vi "Session Reservation Json to Data Cluster.vi"(8 "error in":errorcluster, 11 "json in":string) -> (0 "error out":errorcluster, 3 "data out":T1)   [LabVIEW 2020, in "MeasurementServerTests.lvlib"]
uses:
  MeasurementServerTests.lvlib
  Runtime/MeasurementLink Session Management/Session Reservation/Data.ctl
  Runtime/MeasurementLink Session Management/Connection Map/Connection Map.lvclass
  Runtime/MeasurementLink Session Management/Session Reservation/Session and Driver Info.ctl
  Runtime/MeasurementLink Session Management Client/RPC Messages/ni_measurementlink_sessionmanagement_v1_SessionInformation.ctl
  Runtime/MeasurementLink Session Management Client/RPC Messages/nidevice_grpc_Session.ctl
  Runtime/MeasurementLink Session Management Client/RPC Messages/ni_measurementlink_sessionmanagement_v1_ChannelMapping.ctl
  Runtime/MeasurementLink Session Management Client/RPC Messages/ni_measurementlink_PinMapContext.ctl
  2dfce5ba-96f1-4d0e-9517-3e25601897e8.vi
  <vilib>/JDP Science/JSONtext/JSON text to Variant.vi
  <vilib>/JDP Science/JSONtext/LVClass Serializer/JSONtext LVClass Serializer.lvclass
  Runtime/MeasurementLink Session Management/Session Reservation/Session Reservation.lvclass
  Runtime/MeasurementLink Session Management Client/MeasurementLink Session Management Client.lvlib
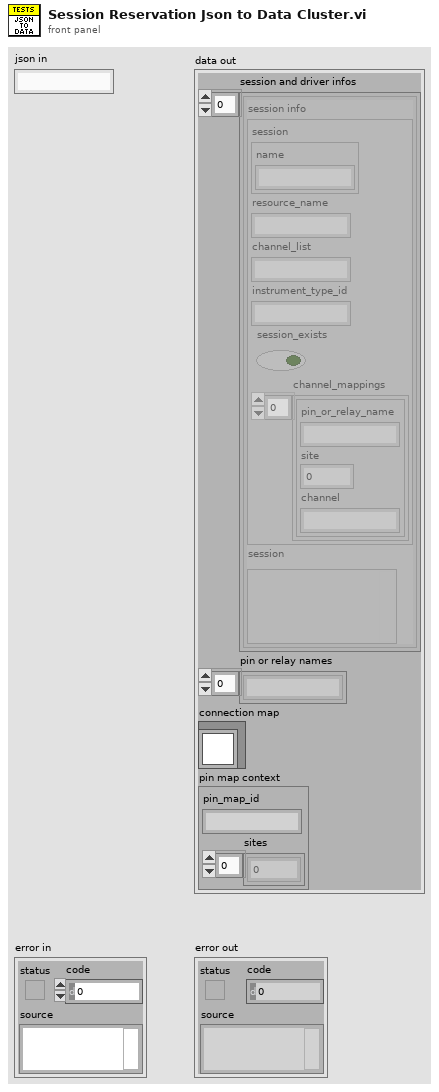
[diagram p1: front panel]
types:
  T1 = typedef "MeasurementLink Session Management.lvlib/Session Reservation.lvclass/Data.ctl" = cluster{"session and driver infos":T2[], "pin or relay names":string[], "connection map":refnum<class "Connection Map.lvclass">, "pin map context":T6}
  T2 = typedef "MeasurementLink Session Management.lvlib/Session Reservation.lvclass/Session and Driver Info.ctl" = cluster{"session info":T3, "session":variant}
  T3 = typedef "MeasurementLink Session Management Client.lvlib/ni_measurementlink_sessionmanagement_v1_SessionInformation.ctl" = cluster{"session":T4, "resource_name":string, "channel_list":string, "instrument_type_id":string, "session_exists":bool, "channel_mappings":T5[]}
  T4 = typedef "MeasurementLink Session Management Client.lvlib/nidevice_grpc_Session.ctl" = cluster{"name":string}
  T5 = typedef "MeasurementLink Session Management Client.lvlib/ni_measurementlink_sessionmanagement_v1_ChannelMapping.ctl" = cluster{"pin_or_relay_name":string, "site":i32, "channel":string}
  T6 = typedef "MeasurementLink Session Management Client.lvlib/ni_measurementlink_PinMapContext.ctl" = cluster{"pin_map_id":string, "sites":i32[]}
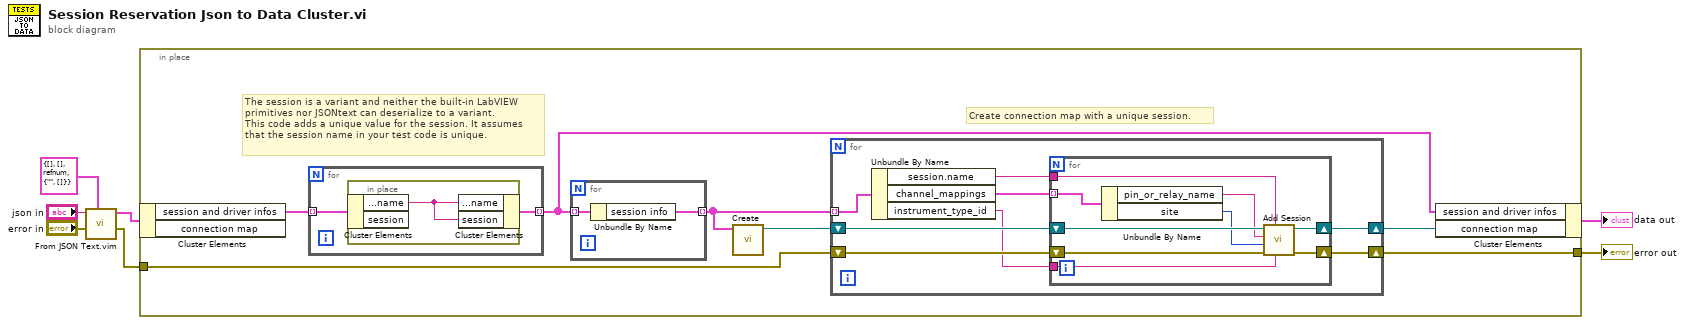
[diagram p0: block diagram]
diagram:
  n1 = call "From JSON Text.vim"("Data Type and Default Value"=T1 {"session and driver infos"=[], "pin or relay names"=[], "connection map"=refnum, "pin map context"={"pin_map_id"="", "sites"=[]}} ("data"), "error in (no error)"="error in", "JSON"="json in") -> ("error out"=w2:errorcluster, "Data out"=w5:T1)  [unwired: 7 in]
  n2 = in-place {
    in-place-border: w2 -> [w12]
    in-place-border: [w11] -> w1
    # "Create connection map with a unique session."
    # "The session is a variant and neither the built-in LabVIEW\nprimitives nor JSONtext can deserialize to a variant.\nThis code adds a unique value for the session. It assumes\nthat the session name in your test code is unique."
    n3 = in-place-cluster #1(w5) -> ("session and driver infos"=w9:T2[])  [unwired: 1 out]
    n4 = for {
      tunnel: w9 -> [w16] mode=indexing
      tunnel: [w15] -> w8 mode=indexing
      n5 = in-place {
        n6 = in-place-cluster #2(w16) -> ("session info.session.name"=w17:string)  [unwired: 1 out]
        n7 = in-place-cluster #2("session info.session.name"=w17, "session"=w17) -> (w15:T2)
      }
    }
    n8 = for {
      tunnel: w8 -> [w36] mode=indexing
      tunnel: [w35] -> w10 mode=indexing
      n9 = Unbundle By Name(w36) -> ("session info"=w35:T3)
    }
    n10 = call "Create.vi"("session info"=w10) -> ("connection map"=w14:refnum<class "Connection Map.lvclass">)  [unwired: 10 in]
    n11 = for {
      shift-right: [w24] -> w13
      shift-left: w14 -> [w25]
      shift-right: [w22] -> w11
      shift-left: w12 -> [w23]
      tunnel: w10 -> [w21] mode=indexing
      n12 = Unbundle By Name(w21) -> ("session.name"=w18:string, "channel_mappings"=w20:T5[], "instrument_type_id"=w19:string)
      n13 = for {
        shift-right: [w33] -> w24
        shift-left: w25 -> [w34]
        shift-right: [w31] -> w22
        shift-left: w23 -> [w32]
        tunnel: w20 -> [w30] mode=indexing
        tunnel: w19 -> [w27]
        tunnel: w18 -> [w26]
        n14 = Unbundle By Name(w30) -> ("pin_or_relay_name"=w29:string, "site"=w28:i32)
        n15 = call "Add Session.vi"("instrument type id"=w27, "session to add"=w26, "error in"=w32, "site"=w28, "pin or relay name"=w29, "connection map in"=w34) -> ("error out"=w31:errorcluster, "connection map out"=w33:refnum<class "Connection Map.lvclass">)  [unwired: 4 in]
      }
    }
    n16 = in-place-cluster #1("session and driver infos"=w8, "connection map"=w13) -> (→"data out":T1)
  }
  "error out" <- w1
